vi "Configure Number of Points.vi"(8 "error in (no error)":errorcluster, 10 "Number of Point":i32, 11 "VNA-ENA in":refnum<class "VNA-ENA.lvclass">) -> (0 "error out":errorcluster, 3 "VNA-ENA out":refnum<class "VNA-ENA.lvclass">)   [LabVIEW 2020, in "VNA-ENA.lvclass"]
doc: "Configures the number of points in the sweep.\nThe number of points will be choosen to the nearest supported."
uses:
  VNA-ENA.lvclass
  C:/Sandbox/RF Bench/Source Code/WiSpry Test Framework/Instruments/Instrument.lvclass
  Instrument.lvclass/Instrument.ctl
  Instrument.lvclass
  <instrlib>/Agilent ENA Series/Agilent ENA Series.lvlib
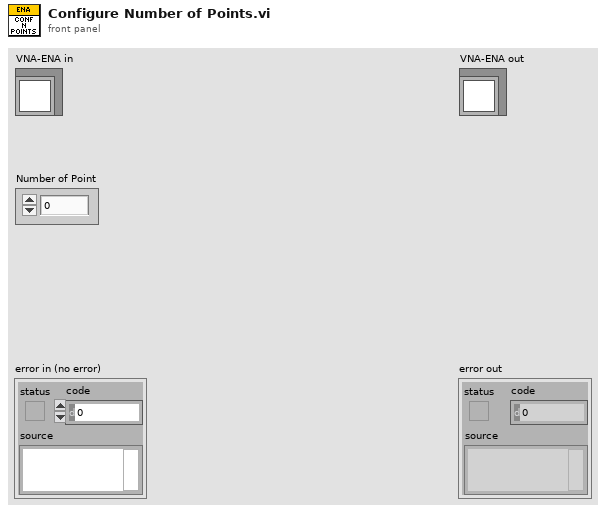
[diagram p1: front panel]
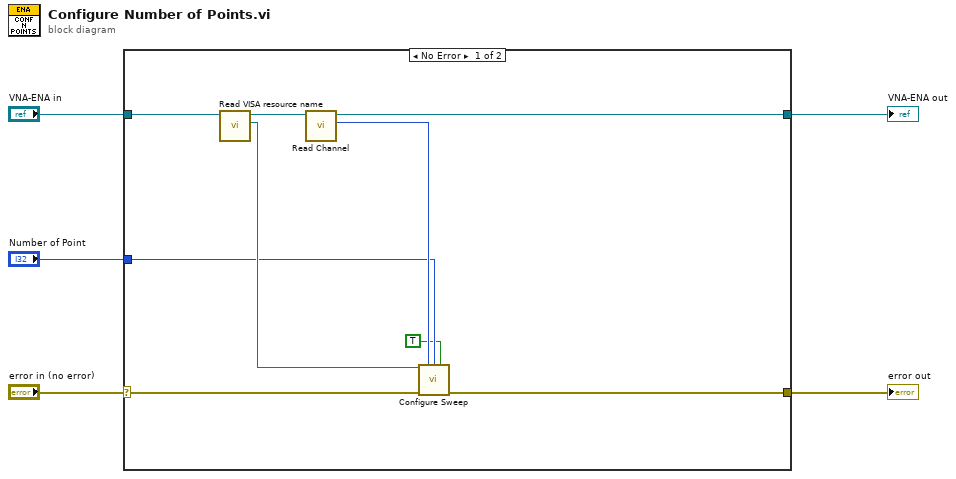
[diagram p0: block diagram]
diagram:
  n1 = case shown="No Error" "error in (no error)" {
    selector: "error in (no error)" -> [w11 w16]
    tunnel: [w10 w16] -> w2
    tunnel: [w13 w15] -> w3
    tunnel: "VNA-ENA in" -> [w14 w15]
    tunnel: "Number of Point" -> [w7 _]
    frame No Error {
      n2 = call "Read VISA resource name.vi"("Instrument in"=w14) -> ("VISA resource name"=w8:refnum<visa-resource-name>, "Instrument out"=w12:refnum<class "VNA-ENA.lvclass">)  [unwired: 9 in]
      n3 = call-dynamic "Read Channel.vi"("Vector Network Analyzer in"=w12) -> ("Channel"=w9:i32, "Vector Network Analyzer out"=w13:refnum<class "VNA-ENA.lvclass">)  [unwired: 9 in]
      n4 = call <instrlib>:"Configure Sweep.vi"("VISA resource name"=w8, "Channel (1)"=w9, "Number of Measurement Points (201)"=w7, "Auto Sweep Time (F: Off)"=TRUE, "error in (no error)"=w11) -> ("error out"=w10:errorcluster)  [unwired: 9 in, 1 out]
    }
    frame Error {
    }
  }
  "error out" <- w2
  "VNA-ENA out" <- w3
